vi "Globals.vi"() -> ()   [LabVIEW 2013, in "GOLPI library.lvlib"]
uses:
  GOLPI library.lvlib
panel:
  in  "fast read to multiple [ms]":u32=1
  in  "fast read settle time [ms]":u32=10
  in  "fast read timeout [ms]":u32=500
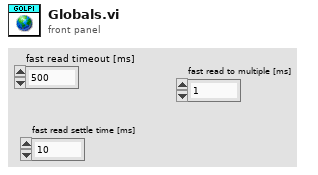
[diagram p1: front panel]
diagram:
